vi "thales_remote_python.vi"() -> ()   [LabVIEW 2023]
panel:
  in  "Target Current":dbl
  in  "IP Address":string
  in  "Potentiostatic/Galvanostatic":bool
  out "Read Voltage":dbl
  out "Read Current":dbl
  in  "Target Voltage":dbl
  out "error out":errorcluster
  in  "error in (no error)":errorcluster
  # "This vi file with the labview_wrapper.py and a Jupyter notebook (.ipynb) with further explanations and documentation can be found on GitHub:\nhttps://github.com/Zahner-elektrik/Thales-Remote-Python/tree/main/Examples/LabVIEW"
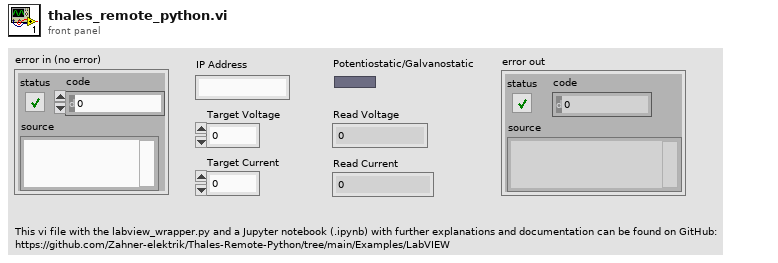
[diagram p1: front panel]
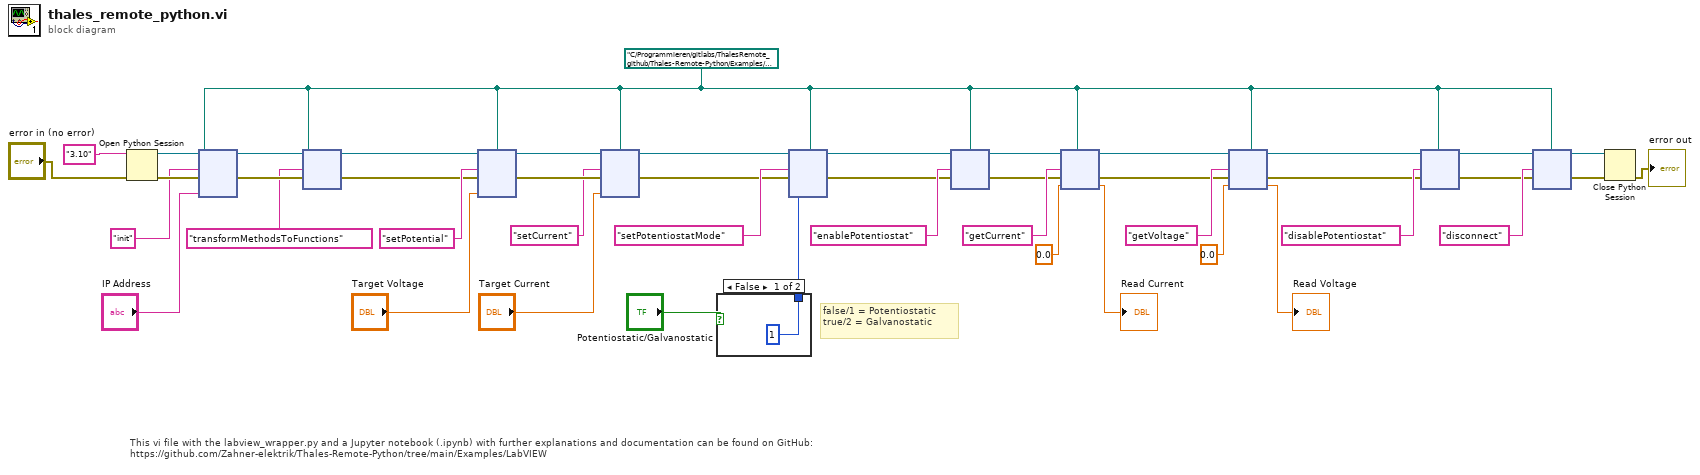
[diagram p0: block diagram]
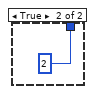
[diagram p2: hidden frame]
diagram:
  w1 = path "C:/Programmieren/gitlabs/ThalesRemote_github/Thales-Remote-Python/Examples/LabVIEW/labview_wrapper.py" ("module path")
  # "This vi file with the labview_wrapper.py and a Jupyter notebook (.ipynb) with further explanations and documentation can be found on GitHub:\nhttps://github.com/Zahner-elektrik/Thales-Remote-Python/tree/main/Examples/LabVIEW"
  # "false/1 = Potentiostatic\ntrue/2 = Galvanostatic"
  n1 = Open Python Session(python version="3.10" ("Python version"), 3:"error in (no error)") -> (session out=w40:refnum<k35>, error out=w42:errorcluster)  [unwired: 1 in]
  n2 = node(w40, w1, "init" ("function name"), w42, "IP Address") -> (w41:refnum<k35>, w43:errorcluster)  [unwired: 3 in, 2 out]
  n3 = node(w41, w1, "transformMethodsToFunctions" ("function name"), w43) -> (w34:refnum<k35>, w32:errorcluster)  [unwired: 2 in, 2 out]
  n4 = node(w34, w1, "setPotential" ("function name"), w32, "Target Voltage") -> (w31:refnum<k35>, w30:errorcluster)  [unwired: 3 in, 2 out]
  n5 = node(w31, w1, "setCurrent" ("function name"), w30, "Target Current") -> (w25:refnum<k35>, w26:errorcluster)  [unwired: 3 in, 2 out]
  n6 = case shown="False" "Potentiostatic/Galvanostatic" {
    tunnel: [1 2] -> w23
    frame False {
    }
    frame True {
    }
  }
  n7 = node(w25, w1, "setPotentiostatMode" ("function name"), w26, w23) -> (w20:refnum<k35>, w21:errorcluster)  [unwired: 3 in, 2 out]
  n8 = node(w20, w1, "enablePotentiostat" ("function name"), w21) -> (w12:refnum<k35>, w11:errorcluster)  [unwired: 2 in, 2 out]
  n9 = node(w12, w1, "getCurrent" ("function name"), w11, 0.0) -> (w9:refnum<k35>, w10:errorcluster, →"Read Current":dbl)  [unwired: 2 out]
  n10 = node(w9, w1, "getVoltage" ("function name"), w10, 0.0) -> (w8:refnum<k35>, w7:errorcluster, →"Read Voltage":dbl)  [unwired: 2 out]
  n11 = node(w8, w1, "disablePotentiostat" ("function name"), w7) -> (w2:refnum<k35>, w5:errorcluster)  [unwired: 2 in, 2 out]
  n12 = node(w2, w1, "disconnect" ("function name"), w5) -> (w3:refnum<k35>, w4:errorcluster)  [unwired: 2 in, 2 out]
  n13 = Close Python Session(session in=w3, error in=w4) -> (11:→"error out":errorcluster)
